vi "recycle logic.vi"(11 "main-national data in":T1) -> (0 "next?":bool, 3 "main-national data out":T1)   [LabVIEW 2019]
uses:
  ctl/main data-national.ctl
  ctl/position set.ctl
panel:
  out "room":string
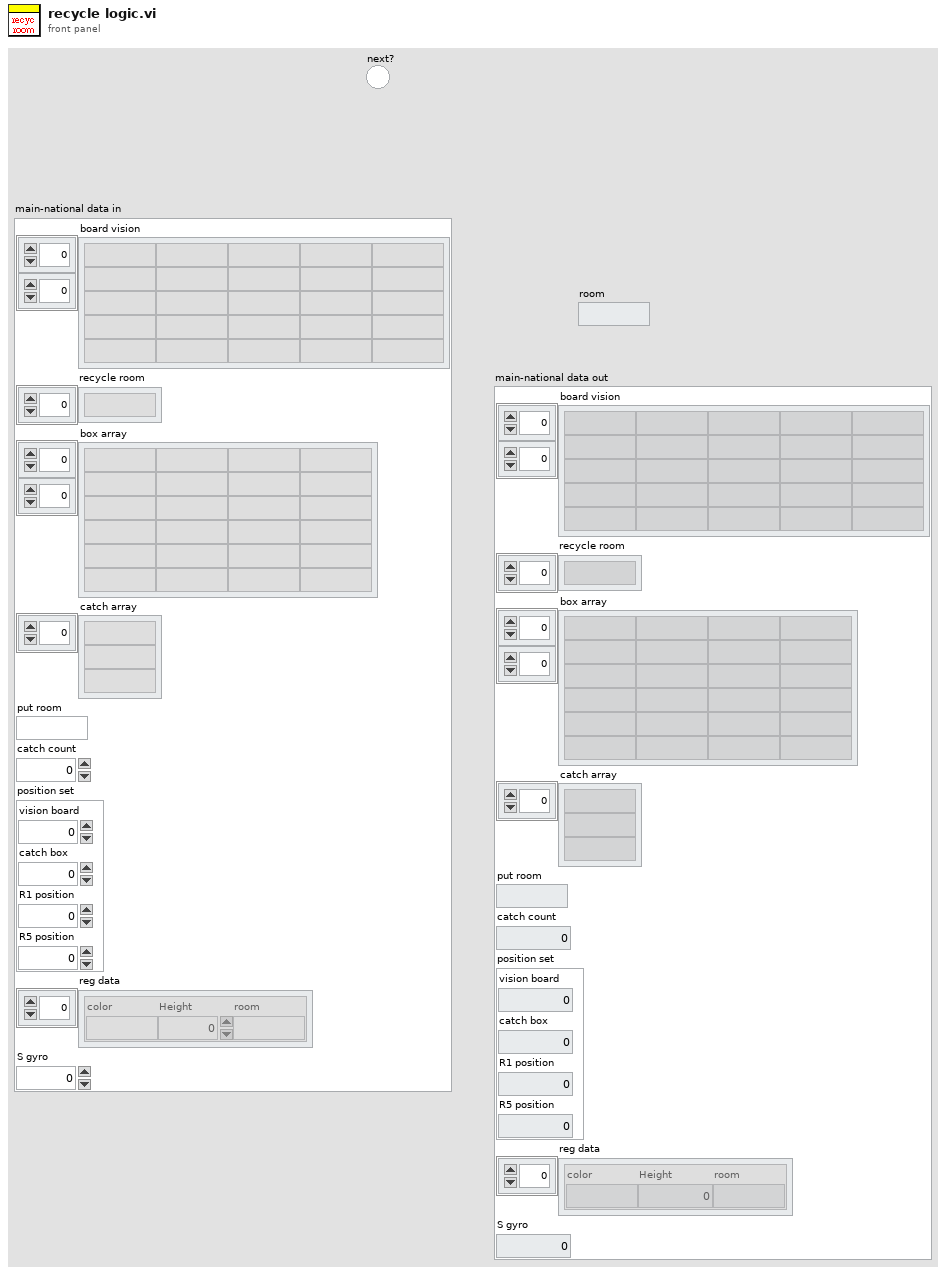
[diagram p1: front panel]
types:
  T1 = typedef "main data-national.ctl" = cluster{"board vision":string[][], "recycle room":string[], "box array":string[][], "catch array":string[], "put room":string, "catch count":dbl, "position set":T2, "reg data":cluster{"color":string, "Height":i32, "room":string}[], "S gyro":dbl}
  T2 = typedef "position set.ctl" = cluster{"vision board":dbl, "catch box":dbl, "R1 position":dbl, "R5 position":dbl}
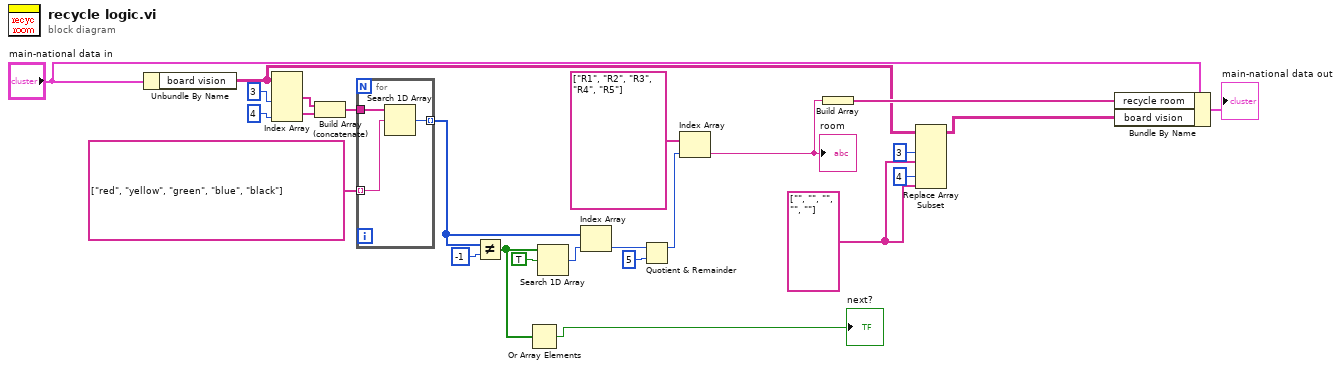
[diagram p0: block diagram]
diagram:
  w5 = string[] ["", "", "", "", ""] ("new element/subarray")
  n1 = Unbundle By Name("main-national data in") -> ("board vision"=w9:string[][])
  n2 = Index Array(array=w9, index (col) #1=3 ("disabled index (col)"), index (col) #2=4 ("index (col)")) -> (element #1=w23:string[], element #2=w22:string[])  [unwired: 2 in]
  n3 = Build Array (concatenate)(w23, w22) -> (w21:string[])
  n4 = for {
    tunnel: w21 -> [w28]
    tunnel: string[] ["red", "yellow", "green", "blue", "black"] -> [w27] mode=indexing
    tunnel: [w26] -> w17 mode=indexing
    n5 = Search 1D Array(1D array=w28, element=w27) -> (index of element=w26:i32)  [unwired: 1 in]
  }
  n6 = Not Equal?(x=w17, y=-1) -> (x != y?=w3:bool[])
  n7 = Or Array Elements(Boolean array=w3) -> (logical OR=→"next?":bool)
  n8 = Search 1D Array(1D array=w3, element=TRUE) -> (index of element=w16:i32)  [unwired: 1 in]
  n9 = Index Array(array=w17, index=w16) -> (element=w15:i32)
  n10 = Quotient & Remainder(x=w15, y=5) -> (x-y*floor(x/y)=w6:i32)  [unwired: 1 out]
  n11 = Index Array(array=string[] ["R1", "R2", "R3", "R4", "R5"], index=w6) -> (element=w1:string)
  "room" <- w1
  n12 = Build Array(w1) -> (w10:string[])
  n13 = Replace Array Subset(array=w9, new element #1=w5, index (col) #1=3 ("disabled index (col)"), new element #2=w5, index (col) #2=4 ("index (col)")) -> (w4:string[][])  [unwired: 2 in]
  n14 = Bundle By Name(cluster="main-national data in", "recycle room"=w10, "board vision"=w4) -> (→"main-national data out":T1)
